vi "Handle Crashed Component Files.vi"(4 "Command Step":dbl, 6 "TemplatePath":path, 7 "Controller List":T2(array[cluster]), 8 "Error In":errorcluster, 10 "[Filenames]":string[](array[string]), 11 "DefaultDataPath":path) -> ()   [LabVIEW 2013]
uses:
  TypeDef/Controller Names.ctl
  <vilib>/Utility/file.llb/Read From Spreadsheet File (string).vi
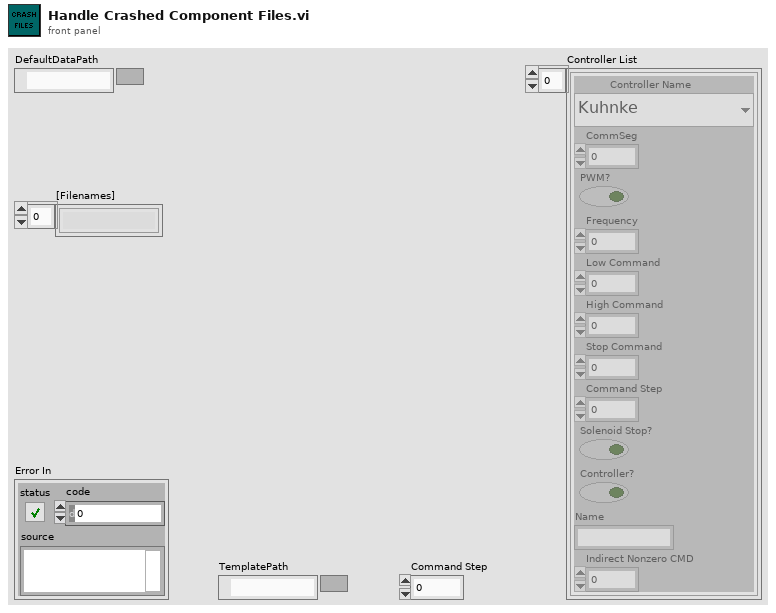
[diagram p1: front panel]
types:
  T1 = typedef "Controller Names.ctl" = enum16{"Kuhnke", "McLaren", "Helbako BLDC", "Conti", "Hella E4LMF", "Hella E4LMD", "Hella E4DCG 20mm", "Hella E4DCG 30mm", "Helbako (old)", "TI PWM", "PSA", "Hella Hyundai Gas", "Hella Hyundai Diesel", "8 Comm", "10 Comm", "8 Comm Hella FCA", "10 Comm Hella FCA", "8 Comm Omron", "10 Comm Omron", "8 Comm Nissan", "10 Comm Nissan"}
  T2 = cluster{"Controller Name":T1, "CommSeg":i32, "PWM?":bool, "Frequency":i32, "Low Command":dbl, "High Command":dbl, "Stop Command":dbl, "Command Step":dbl, "Solenoid Stop?":bool, "Controller?":bool, "Name":string, "Indirect Nonzero CMD":dbl}[]
  T3 = cluster{"appended path":path, bool, "TestType":enum32{"Flow", "Timed", "Hot\nFuel"}}
  T4 = cluster{"appended path":path, bool, "TestType":enum32{"Flow", "Timed", "Hot\nFuel"}}[]
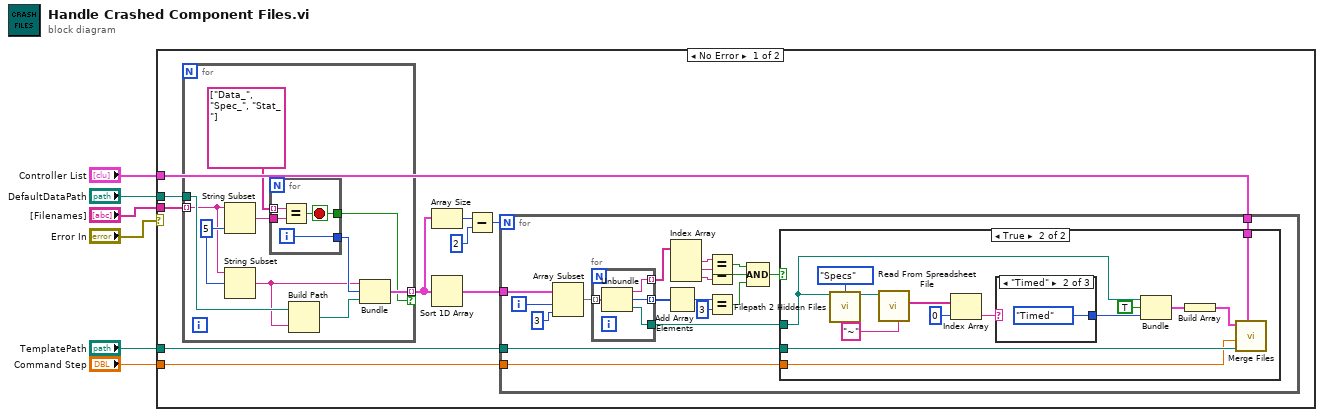
[diagram p0: block diagram]
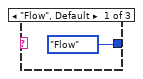
[diagram p3: hidden frame]
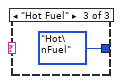
[diagram p4: hidden frame]
diagram:
  n1 = case shown="No Error" "Error In" {
    tunnel: "DefaultDataPath" -> [w16 _]
    tunnel: "[Filenames]" -> [w15 _]
    tunnel: "TemplatePath" -> [w9 _]
    tunnel: "Controller List" -> [w8 _]
    tunnel: "Command Step" -> [w7 _]
    frame No Error {
      n2 = for {
        tunnel: w16 -> [w64]
        tunnel: w15 -> [w58] mode=indexing
        tunnel: [w61] -> w14 mode=indexing if=w60
        w63 = 5 ("length (rest)")
        n3 = String Subset(string=w58, length (rest)=w63) -> (substring=w66:string)  [unwired: 1 in]
        n4 = String Subset(string=w58, offset (0)=w63) -> (substring=w57:string)  [unwired: 1 in]
        n5 = for {
          tunnel: w66 -> [w69]
          tunnel: string[] ["Data_", "Spec_", "Stat_"] -> [w70] mode=indexing
          tunnel: [w68] -> w60
          tunnel: [w67] -> w62
          i -> [w67]
          stop <- w68 stop-if-true
          n6 = Equal?(x=w70, y=w69) -> (x = y?=w68:bool)
        }
        n7 = Build Path(base path=w64, name or relative path=w57) -> (appended path=w59:path)
        n8 = Bundle(w57, w62, "appended path"=w59) -> (w61:cluster{string, i32, "appended path":path})  [unwired: 1 in]
      }
      n9 = Array Size(array=w14) -> (size(s)=w12:i32)
      n10 = Sort 1D Array(array=w14) -> (sorted array=w13:cluster{string, i32, "appended path":path}[])
      n11 = Subtract(x=w12, y=2) -> (x-y=w10:i32)
      n12 = for {
        N: w10 -> [_]
        tunnel: w13 -> [w35]
        tunnel: w9 -> [w19]
        tunnel: w8 -> [w18]
        tunnel: w7 -> [w17]
        i -> [w34]
        n13 = Array Subset(array=w35, index=w34, length=3) -> (w32:cluster{string, i32, "appended path":path}[])
        n14 = for {
          tunnel: w32 -> [w56] mode=indexing
          tunnel: [w55] -> w31 mode=indexing
          tunnel: [w54] -> w30 mode=indexing
          tunnel: [w53] -> w20
          n15 = Unbundle(w56) -> (w54:string, w55:i32, "appended path"=w53:path)
        }
        n16 = Add Array Elements(numeric array=w31) -> (sum=w26:i32)
        n17 = Index Array(array=w30) -> (element #1=w28:string, element #2=w29:string, element #3=w27:string)  [unwired: 3 in]
        n18 = Equal?(x=w28, y=w29) -> (x = y?=w24:bool)
        n19 = Equal?(x=w29, y=w27) -> (x = y?=w23:bool)
        n20 = Equal?(x=w26, y=3) -> (x = y?=w22:bool)
        n21 = Compound Arithmetic op=AND(w24, w23, w22) -> (w21:bool)
        n22 = case shown="True" w21 {
          tunnel: w20 -> [_ w36]
          tunnel: w19 -> [_ w48]
          tunnel: w18 -> [_ w45]
          tunnel: w17 -> [_ w44]
          frame False {
          }
          frame True {
            n23 = call "Filepath 2 Hidden Files.vi"("DataFilePath"=w36, "Enum"=enum16{"Data", "Stats", "Specs"}."Specs") -> ("HiddenFilePath"=w43:path)  [unwired: 13 in]
            n24 = call-poly <vilib>:"Read From Spreadsheet File.vi"("delimiter (\\t)"="~" ("delimiter (\\t)"), "file path (dialog if empty)"=w43) -> ("first row"=w41:string[])  [unwired: 5 in, 4 out]
            n25 = Index Array(array=w41, index=0 ("index (row)")) -> (element=w42:string)
            n26 = case shown="\"Timed\"" w42 {
              tunnel: [enum32{"Flow", "Timed", "Hot\nFuel"}."Flow" ("TestType") enum32{"Flow", "Timed", "Hot\nFuel"}."Timed" ("TestType") enum32{"Flow", "Timed", "Hot\nFuel"}."Hot\nFuel" ("TestType")] -> w37
              frame "Flow", Default {
              }
              frame "Timed" {
              }
              frame "Hot Fuel" {
              }
            }
            n27 = Bundle("appended path"=w36, TRUE, "TestType"=w37) -> (w46:T3)  [unwired: 1 in]
            n28 = Build Array(w46) -> (w49:T4)
            n29 = call "Merge Files.vi"("Controller List"=w45, "TemplatePath"=w48, "CMD Step"=w44, "Created/ModFiles"=w49) -> ()  [unwired: 8 in]
          }
        }
      }
    }
    frame Error {
    }
  }
